vi "SetWavelength_175.vi"(8 "error in":errorcluster, 9 "wavelength":dbl, 10 "Slit":string, 11 "Port":refnum<visa-resource-name>) -> (0 "error out":errorcluster, 3 "Port out":refnum<visa-resource-name>)   [LabVIEW 2018]
panel:
  out "Final response":u8
  out "Response":u8
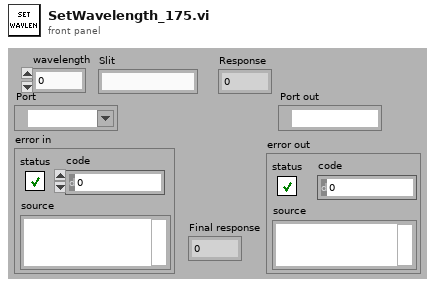
[diagram p1: front panel]
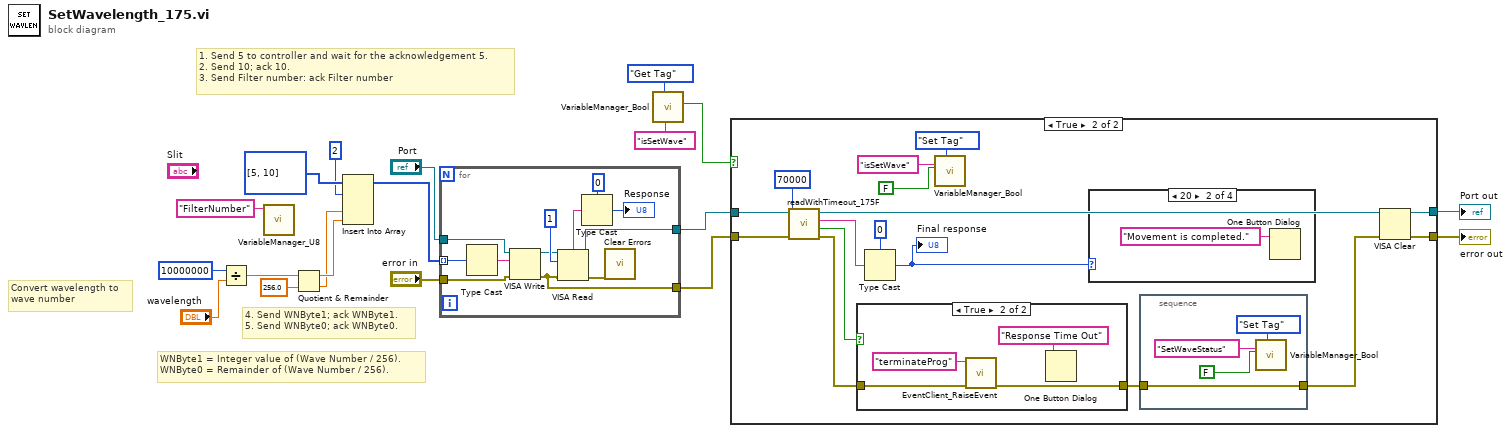
[diagram p0: block diagram]
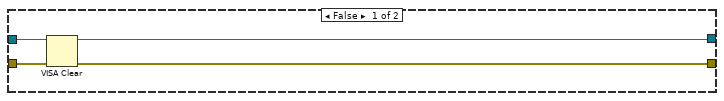
[diagram p2: hidden frame]
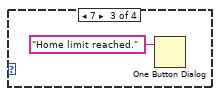
[diagram p5: hidden frame]
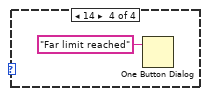
[diagram p6: hidden frame]
diagram:
  # "WNByte1 = Integer value of (Wave Number / 256).\nWNByte0 = Remainder of (Wave Number / 256)."
  # "4. Send WNByte1; ack WNByte1.\n5. Send WNByte0; ack WNByte0."
  # "1. Send 5 to controller and wait for the acknowledgement 5.\n2. Send 10; ack 10.\n3. Send Filter number: ack Filter number"
  # "Convert wavelength to\nwave number"
  n1 = Divide(x=u32 10000000 ("timeOut"), y="wavelength") -> (x/y=w14:dbl)
  n2 = call "VariableManager_U8.vi"("Tag"="FilterNumber") -> ()  [unwired: 7 in, 4 out]
  n3 = Quotient & Remainder(x=w14, y=256.0) -> (x-y*floor(x/y)=w9:dbl, floor(x/y)=w8:dbl)
  n4 = Insert Into Array(array=u8[] [5, 10], index=2, new element #2=w8, new element #3=w9) -> (w11:u8[])  [unwired: 1 in]
  n5 = for {
    tunnel: "Port" -> [w31]
    tunnel: "error in" -> [w30]
    tunnel: [w20] -> w1
    tunnel: [w24] -> w2
    tunnel: w11 -> [w28] mode=indexing
    n6 = Type Cast(x=w28) -> (*(type *) &x=w29:string)  [unwired: 1 in]
    n7 = VISA Write(VISA resource name=w31, write buffer=w29, error in (no error)=w30) -> (VISA resource name out=w22:refnum<visa-resource-name>, error out=w20:errorcluster)  [unwired: 1 out]
    n8 = VISA Read(VISA resource name=w22, byte count=u32 1 ("timeOut"), error in (no error)=w20) -> (VISA resource name out=w24:refnum<visa-resource-name>, read buffer=w25:string, error out=w21:errorcluster)  [unwired: 1 out]
    n9 = Type Cast(type=u8 0 ("timeOut"), x=w25) -> (*(type *) &x=→"Response":u8)
    n10 = call <vilib>:"Clear Errors.vi"("error in (no error)"=w21) -> ()  [unwired: 5 in, 2 out]
  }
  n11 = call "VariableManager_Bool.vi"("Operation"=enum16{"Get Tag", "Set Tag"}."Get Tag", "Tag"="isSetWave") -> ("Value out"=w5:bool)  [unwired: 6 in, 3 out]
  n12 = case shown="True" w5 {
    tunnel: [w35 w38] -> w4
    tunnel: [w33 w36] -> w3
    tunnel: w2 -> [w34 w43]
    tunnel: w1 -> [w32 w42]
    frame False {
      n13 = VISA Clear(VISA resource name=w34, error in (no error)=w32) -> (VISA resource name out=w35:refnum<visa-resource-name>, error out=w33:errorcluster)
    }
    frame True {
      n14 = call "readWithTimeout_175F.vi"("error in"=w42, "timeOut"=u32 70000, "Port"=w43) -> ("error out"=w41:errorcluster, "TimeOut"=w44:bool, "String"=w47:string, "Port out"=w39:refnum<visa-resource-name>)  [unwired: 5 in]
      n15 = case shown="True" w44 {
        tunnel: [w56 w58] -> w40
        tunnel: w41 -> [w56 w57]
        frame False {
        }
        frame True {
          n16 = call "EventClient_RaiseEvent.vi"("error in (no error)"=w57, "Event"="terminateProg") -> ("error out"=w58:errorcluster)  [unwired: 9 in]
          n17 = One Button Dialog(message="Response Time Out") -> ()  [unwired: 1 in, 1 out]
        }
      }
      n18 = Type Cast(type=u8 0 ("timeOut"), x=w47) -> (*(type *) &x=w45:u8)
      "Final response" <- w45
      n19 = call "VariableManager_Bool.vi"("Operation"=enum16{"Get Tag", "Set Tag"}."Set Tag", "Value"=FALSE, "Tag"="isSetWave") -> ()  [unwired: 5 in, 4 out]
      n20 = case shown="20" w45 {
        frame 0, Default {
        }
        frame 20 {
          n21 = One Button Dialog(message="Movement is completed.") -> ()  [unwired: 1 in, 1 out]
        }
        frame 7 {
          n22 = One Button Dialog(message="Home limit reached.") -> ()  [unwired: 1 in, 1 out]
        }
        frame 14 {
          n23 = One Button Dialog(message="Far limit reached") -> ()  [unwired: 1 in, 1 out]
        }
      }
      n24 = stacked-sequence {
        tunnel: [w55] -> w37
        tunnel: w40 -> [w55]
        frame #0 {
          n25 = call "VariableManager_Bool.vi"("Operation"=enum16{"Get Tag", "Set Tag"}."Set Tag", "Value"=FALSE, "Tag"="SetWaveStatus") -> ()  [unwired: 5 in, 4 out]
        }
      }
      n26 = VISA Clear(VISA resource name=w39, error in (no error)=w37) -> (VISA resource name out=w38:refnum<visa-resource-name>, error out=w36:errorcluster)
    }
  }
  "Port out" <- w4
  "error out" <- w3
